vi "Bridge2_Main.vi"() -> (0 "error out":errorcluster)   [LabVIEW 2020]
uses:
  IEnchantment_interface/IEnchantment.lvclass
  FlyingEnchantment_class/FlyingEnchantment.lvclass
  C:/Projects/DesignPatterns/Bridge2/IEnchantment_interface/IEnchantment.lvclass
  SoulEatingEnchantment_class/SoulEatingEnchantment.lvclass
  Sword_class/Sword.lvclass
  Hammer_class/Hammer.lvclass
  Console_class/Console.lvclass
panel:
  in  "Add Some Flying Enchantment":bool
  out "TextOut":string
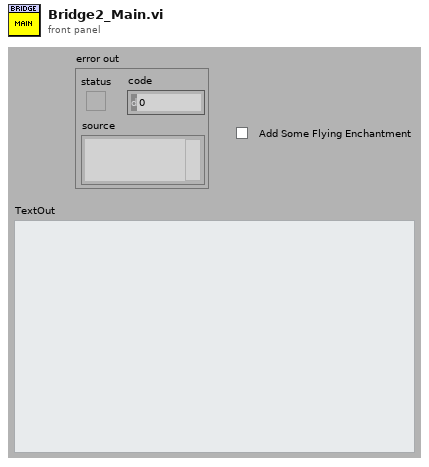
[diagram p1: front panel]
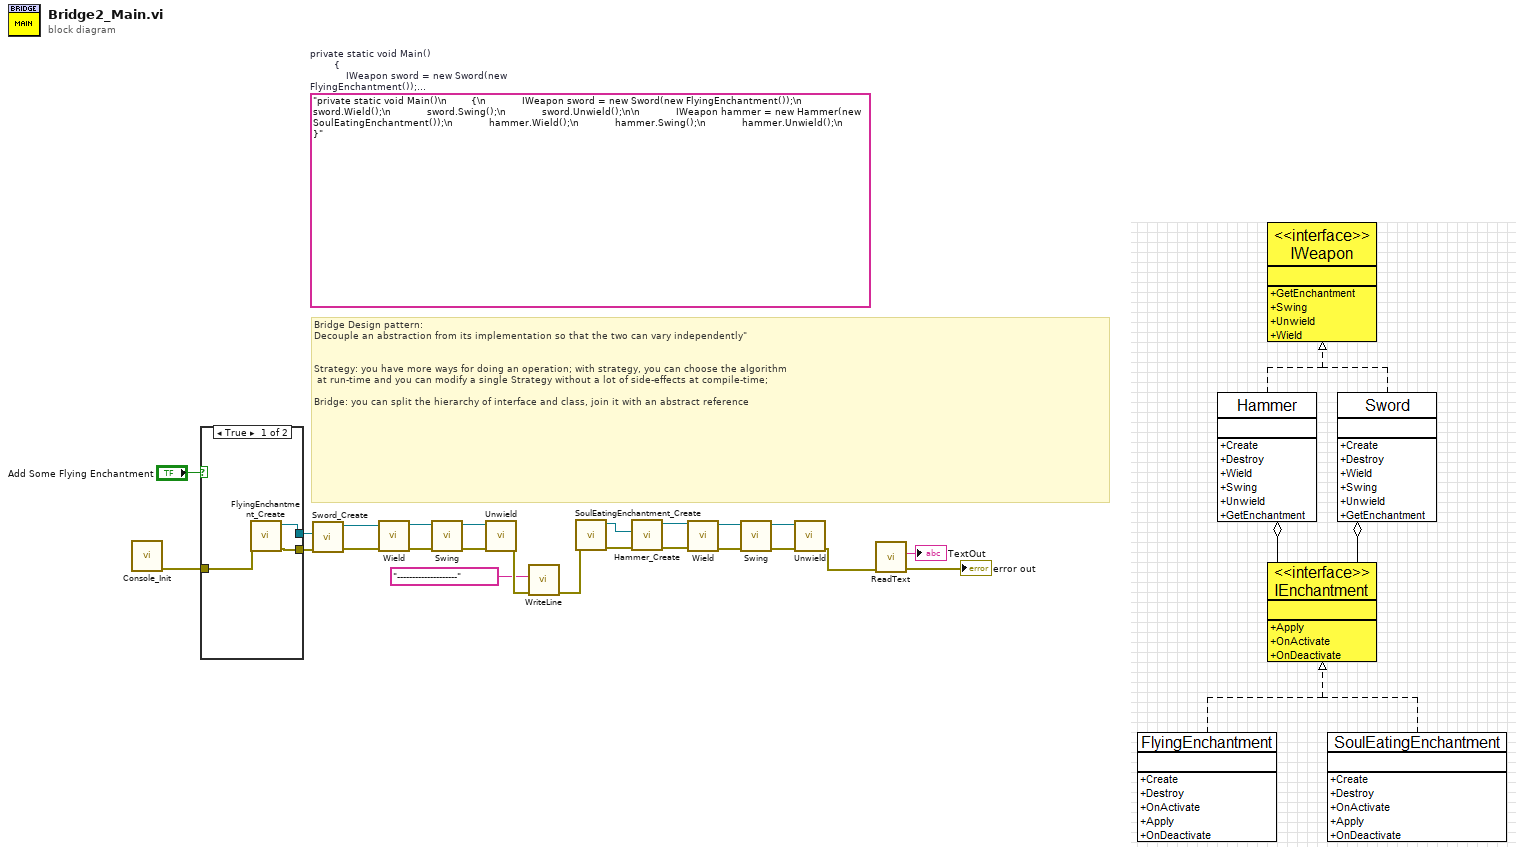
[diagram p0: block diagram]
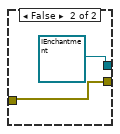
[diagram p2: hidden frame]
diagram:
  (unwired) "private static void Main()\n        {\n            IWeapon sword = new Sword(new FlyingEnchantment());\n            sword.Wield();\n            sword.Swing();\n            sword.Unwield();\n\n            IWeapon hammer = new Hammer(new SoulEatingEnchantment());\n            hammer.Wield();\n            hammer.Swing();\n            hammer.Unwield();\n        }"  # private static void Main()         {             IWeapon sword = new Sword(new FlyingEnchantment());             sword.Wield();             sword.Swing();             sword.Unwield();              IWeapon hammer = new Hammer(new SoulEatingEnchantment());             hammer.Wield();             hammer.Swing();             hammer.Unwield();         }
  # "Bridge Design pattern:\nDecouple an abstraction from its implementation so that the two can vary independently\"\n\n\nStrategy: you have more ways for doing an operation; with strategy, you can choose the algorithm\n at run-time and you can modify a single Strategy without a lot of side-effects at compile-time;\n\nBridge: you can split the hierarchy of interface and class, join it with an abstract reference"
  n1 = call "Console_Init.vi"() -> ("Error Out"=w8:errorcluster)  [unwired: 10 in, 1 out]
  n2 = case shown="True" "Add Some Flying Enchantment" {
    tunnel: [w27 refnum<class "IEnchantment.lvclass"> refnum ("IEnchantment")] -> w23
    tunnel: [w26 w28] -> w22
    tunnel: w8 -> [w25 w28]
    frame True {
      n3 = call "FlyingEnchantment_Create.vi"("Error In"=w25) -> ("Error Out"=w26:errorcluster, "reference out"=w27:refnum<class "FlyingEnchantment.lvclass">)  [unwired: 9 in]
    }
    frame False {
    }
  }
  n4 = call "Sword_Create.vi"("Error In"=w22, "Enchantment"=w23) -> ("Error Out"=w20:errorcluster, "reference out"=w21:refnum<class "Sword.lvclass">)  [unwired: 8 in]
  n5 = call-dynamic "Wield.vi"("Error In"=w20, "reference in"=w21) -> ("Error Out"=w17:errorcluster, "reference out"=w18:refnum<class "Sword.lvclass">)  [unwired: 8 in]
  n6 = call-dynamic "Swing.vi"("Error In"=w17, "reference in"=w18) -> ("Error Out"=w16:errorcluster, "reference out"=w19:refnum<class "Sword.lvclass">)  [unwired: 8 in]
  n7 = call-dynamic "Unwield.vi"("Error In"=w16, "reference in"=w19) -> ("Error Out"=w4:errorcluster)  [unwired: 8 in, 1 out]
  n8 = call "WriteLine.vi"("Error In"=w4, "ConsoleText"="--------------------") -> ("Error Out"=w3:errorcluster)  [unwired: 9 in]
  n9 = call "SoulEatingEnchantment_Create.vi"("Error In"=w3) -> ("Error Out"=w15:errorcluster, "reference out"=w6:refnum<class "SoulEatingEnchantment.lvclass">)  [unwired: 9 in]
  n10 = call "Hammer_Create.vi"("Error In"=w15, "Enchantment"=w6) -> ("Error Out"=w12:errorcluster, "reference out"=w11:refnum<class "Hammer.lvclass">)  [unwired: 8 in]
  n11 = call-dynamic "Wield.vi"("Error In"=w12, "reference in"=w11) -> ("Error Out"=w10:errorcluster, "reference out"=w14:refnum<class "Hammer.lvclass">)  [unwired: 8 in]
  n12 = call-dynamic "Swing.vi"("Error In"=w10, "reference in"=w14) -> ("Error Out"=w9:errorcluster, "reference out"=w13:refnum<class "Hammer.lvclass">)  [unwired: 8 in]
  n13 = call-dynamic "Unwield.vi"("Error In"=w9, "reference in"=w13) -> ("Error Out"=w7:errorcluster)  [unwired: 8 in, 1 out]
  n14 = call "ReadText.vi"("Error In"=w7) -> ("Error Out"=→"error out":errorcluster, "TextOut"=→"TextOut":string)  [unwired: 9 in]
